vi "Toggle Unit Test CDS.vi"(8 "error in (no error)":errorcluster, 11 "Requested State":bool) -> (0 "error out":errorcluster)   [LabVIEW 2016]
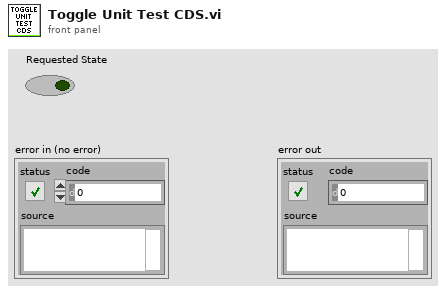
[diagram p1: front panel]
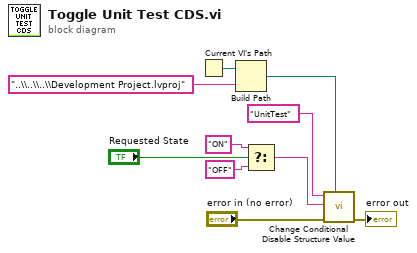
[diagram p0: block diagram]
diagram:
  n1 = Current VI's Path() -> (path=w3:path)
  n2 = Build Path(base path=w3, name or relative path="..\\..\\..\\Development Project.lvproj") -> (appended path=w1:path)
  n3 = Select(t="ON" ("Requested Value"), s="Requested State", f="OFF") -> (s? t:f=w5:string)
  n4 = call "Change Conditional Disable Structure Value.vi"("Project Path"=w1, "error in (no error)"="error in (no error)", "Requested Value"=w5, "Flag to find"="UnitTest") -> ("error out"=→"error out":errorcluster)  [unwired: 6 in, 1 out]
